vi "Config-Sweep-Sync Sour.vi"(6 "power compliance (0 = OFF)":dbl format="%^.2e", 7 "compliance":dbl=2.0 format="%^.2e", 8 "error in (no error)":errorcluster, 9 "ratio":dbl=1.0 format="%^.2e", 10 "offset":dbl=1.2333 format="%^.4e", 11 "VISA session":refnum<visa-resource-name>) -> (0 "error out":errorcluster, 3 "VISA resource name out":refnum<visa-resource-name>)   [LabVIEW 2016, in "Agilent 415X Series.lvlib"]
doc: "This VI configures the synchronous sweep source (VAR1') for a sweep mode measurement.\n \n* This VI does not perform error checking on MEASUREMENT MODE or UNIT TYPE of VAR2, therefore it is the application programmer's responsibility to make certain this VI is used in the proper mode.\n\n** This VI should be used only when a synchronous source is specified."
uses:
  Agilent 415X Series.lvlib
panel:
  # "This VI should be used only when a synchronous\nsource (SMU or VSU) is specified."
  # "(W)"
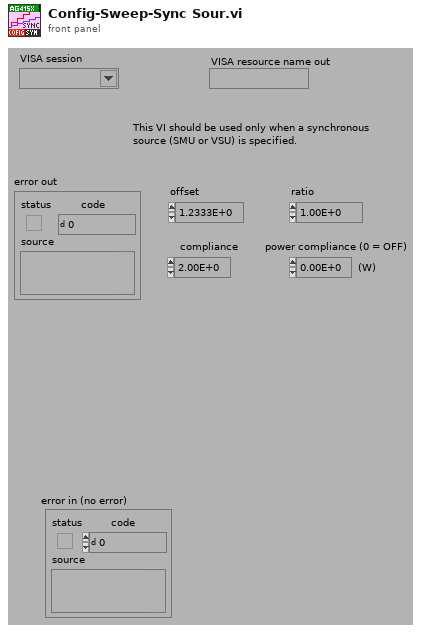
[diagram p1: front panel]
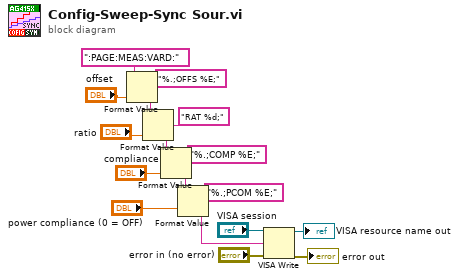
[diagram p0: block diagram]
diagram:
  n1 = Format Value(string ("")=":PAGE:MEAS:VARD:", format string="%.;OFFS %E;", value (0)="offset") -> (output string=w14:string)
  n2 = Format Value(string ("")=w14, format string="RAT %d;", value (0)="ratio") -> (output string=w2:string)
  n3 = Format Value(string ("")=w2, format string="%.;COMP %E;", value (0)="compliance") -> (output string=w3:string)
  n4 = Format Value(string ("")=w3, format string="%.;PCOM %E;", value (0)="power compliance (0 = OFF)") -> (output string=w9:string)
  n5 = VISA Write(VISA resource name="VISA session", write buffer=w9, error in (no error)="error in (no error)") -> (VISA resource name out=→"VISA resource name out":refnum<visa-resource-name>, error out=→"error out":errorcluster)  [unwired: 1 out]
